vi "1A Helper - LatLong ddmm.mm to dd.dddd.vi"(1 "Lattitude/Longitude in ddmm.mmmm":dbl) -> (0 "Latitude/Longitude in dd.dddddd":dbl)   [LabVIEW 2013]
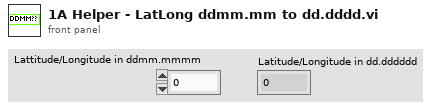
[diagram p1: front panel]
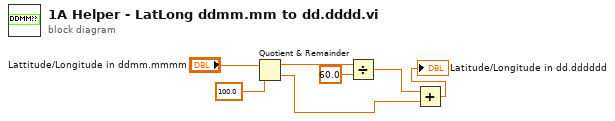
[diagram p0: block diagram]
diagram:
  n1 = Quotient & Remainder(x="Lattitude/Longitude in ddmm.mmmm", y=100.0) -> (x-y*floor(x/y)=w5:dbl, floor(x/y)=w1:dbl)
  n2 = Divide(x=w5, y=60.0) -> (x/y=w2:dbl)
  n3 = Add(x=w2, y=w1) -> (x+y=→"Latitude/Longitude in dd.dddddd":dbl)
